vi "Read_OPC_Stroke.vi"(4 "Test Name":string(combo)="ST1_WL") -> (0 "Stroke_Min":u16, 2 "Stroke_Max":u16)   [LabVIEW 2017]
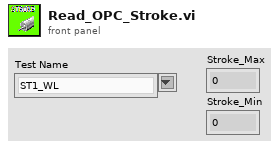
[diagram p1: front panel]
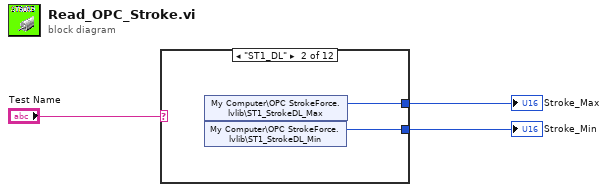
[diagram p0: block diagram]
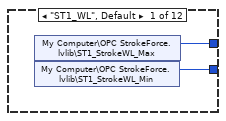
[diagram p2: hidden frame]
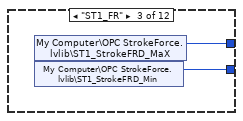
[diagram p3: hidden frame]
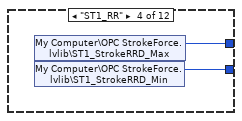
[diagram p4: hidden frame]
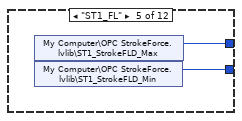
[diagram p5: hidden frame]
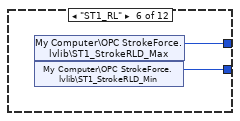
[diagram p6: hidden frame]
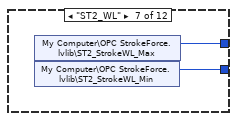
[diagram p7: hidden frame]
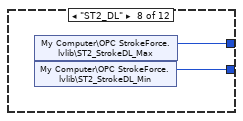
[diagram p8: hidden frame]
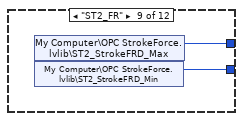
[diagram p9: hidden frame]
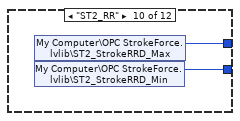
[diagram p10: hidden frame]
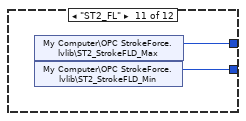
[diagram p11: hidden frame]
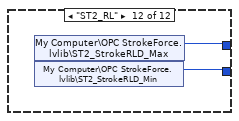
[diagram p12: hidden frame]
diagram:
  n1 = case shown="\"ST1_DL\"" "Test Name" {
    tunnel: [w5 w7 w9 w11 w13 w15 w17 w19 w21 w23 w25 w27] -> w2
    tunnel: [w4 w6 w8 w10 w12 w14 w16 w18 w20 w22 w24 w26] -> w1
    frame "ST1_WL", Default {
      n2 = shared-variable "My Computer\\OPC StrokeForce.lvlib\\ST1_StrokeWL_Max"() -> (w5:u16)  [unwired: 1 in, 1 out]
      n3 = shared-variable "My Computer\\OPC StrokeForce.lvlib\\ST1_StrokeWL_Min"() -> (w4:u16)  [unwired: 1 in, 1 out]
    }
    frame "ST1_DL" {
      n4 = shared-variable "My Computer\\OPC StrokeForce.lvlib\\ST1_StrokeDL_Max"() -> (w7:u16)  [unwired: 1 in, 1 out]
      n5 = shared-variable "My Computer\\OPC StrokeForce.lvlib\\ST1_StrokeDL_Min"() -> (w6:u16)  [unwired: 1 in, 1 out]
    }
    frame "ST1_FR" {
      n6 = shared-variable "My Computer\\OPC StrokeForce.lvlib\\ST1_StrokeFRD_MaX"() -> (w9:u16)  [unwired: 1 in, 1 out]
      n7 = shared-variable "My Computer\\OPC StrokeForce.lvlib\\ST1_StrokeFRD_Min"() -> (w8:u16)  [unwired: 1 in, 1 out]
    }
    frame "ST1_RR" {
      n8 = shared-variable "My Computer\\OPC StrokeForce.lvlib\\ST1_StrokeRRD_Max"() -> (w11:u16)  [unwired: 1 in, 1 out]
      n9 = shared-variable "My Computer\\OPC StrokeForce.lvlib\\ST1_StrokeRRD_Min"() -> (w10:u16)  [unwired: 1 in, 1 out]
    }
    frame "ST1_FL" {
      n10 = shared-variable "My Computer\\OPC StrokeForce.lvlib\\ST1_StrokeFLD_Max"() -> (w13:u16)  [unwired: 1 in, 1 out]
      n11 = shared-variable "My Computer\\OPC StrokeForce.lvlib\\ST1_StrokeFLD_Min"() -> (w12:u16)  [unwired: 1 in, 1 out]
    }
    frame "ST1_RL" {
      n12 = shared-variable "My Computer\\OPC StrokeForce.lvlib\\ST1_StrokeRLD_Max"() -> (w15:u16)  [unwired: 1 in, 1 out]
      n13 = shared-variable "My Computer\\OPC StrokeForce.lvlib\\ST1_StrokeRLD_Min"() -> (w14:u16)  [unwired: 1 in, 1 out]
    }
    frame "ST2_WL" {
      n14 = shared-variable "My Computer\\OPC StrokeForce.lvlib\\ST2_StrokeWL_Max"() -> (w17:u16)  [unwired: 1 in, 1 out]
      n15 = shared-variable "My Computer\\OPC StrokeForce.lvlib\\ST2_StrokeWL_Min"() -> (w16:u16)  [unwired: 1 in, 1 out]
    }
    frame "ST2_DL" {
      n16 = shared-variable "My Computer\\OPC StrokeForce.lvlib\\ST2_StrokeDL_Max"() -> (w19:u16)  [unwired: 1 in, 1 out]
      n17 = shared-variable "My Computer\\OPC StrokeForce.lvlib\\ST2_StrokeDL_Min"() -> (w18:u16)  [unwired: 1 in, 1 out]
    }
    frame "ST2_FR" {
      n18 = shared-variable "My Computer\\OPC StrokeForce.lvlib\\ST2_StrokeFRD_Max"() -> (w21:u16)  [unwired: 1 in, 1 out]
      n19 = shared-variable "My Computer\\OPC StrokeForce.lvlib\\ST2_StrokeFRD_Min"() -> (w20:u16)  [unwired: 1 in, 1 out]
    }
    frame "ST2_RR" {
      n20 = shared-variable "My Computer\\OPC StrokeForce.lvlib\\ST2_StrokeRRD_Max"() -> (w23:u16)  [unwired: 1 in, 1 out]
      n21 = shared-variable "My Computer\\OPC StrokeForce.lvlib\\ST2_StrokeRRD_Min"() -> (w22:u16)  [unwired: 1 in, 1 out]
    }
    frame "ST2_FL" {
      n22 = shared-variable "My Computer\\OPC StrokeForce.lvlib\\ST2_StrokeFLD_Max"() -> (w25:u16)  [unwired: 1 in, 1 out]
      n23 = shared-variable "My Computer\\OPC StrokeForce.lvlib\\ST2_StrokeFLD_Min"() -> (w24:u16)  [unwired: 1 in, 1 out]
    }
    frame "ST2_RL" {
      n24 = shared-variable "My Computer\\OPC StrokeForce.lvlib\\ST2_StrokeRLD_Max"() -> (w27:u16)  [unwired: 1 in, 1 out]
      n25 = shared-variable "My Computer\\OPC StrokeForce.lvlib\\ST2_StrokeRLD_Min"() -> (w26:u16)  [unwired: 1 in, 1 out]
    }
  }
  "Stroke_Max" <- w2
  "Stroke_Min" <- w1
